vi "In.vi"(8 "错误输入":errorcluster caption="错误输入（无错误）", 9 "数据":variant, 10 "指令":string="选择语言", 11 "队列":refnum<queue>) -> (0 "错误输出":errorcluster, 3 "队列输出":refnum<queue>)   [LabVIEW 2020]
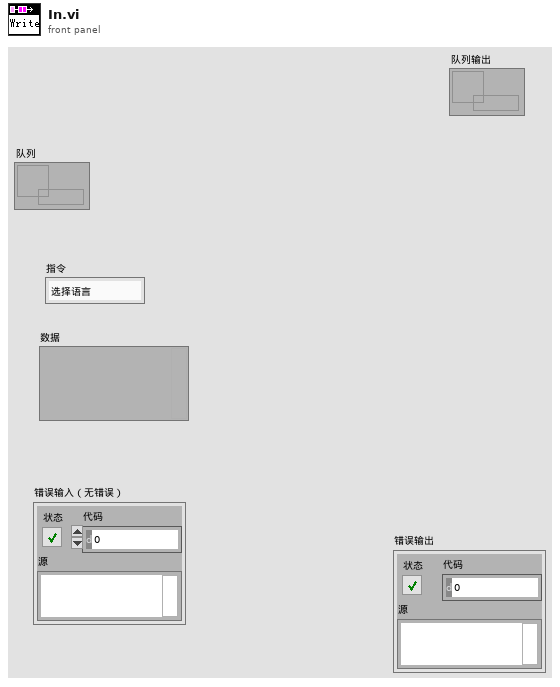
[diagram p1: front panel]
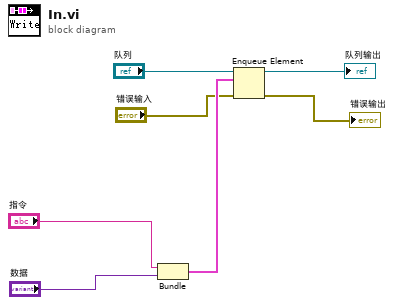
[diagram p0: block diagram]
diagram:
  n1 = Bundle("指令"="指令", "数据"="数据") -> (w6:cluster{"指令":string, "数据":variant})  [unwired: 1 in]
  n2 = Enqueue Element(queue="队列", element=w6, error in (no error)="错误输入") -> (queue out=→"队列输出":refnum<queue>, error out=→"错误输出":errorcluster)  [unwired: 1 in, 1 out]
